vi "Stop Core.vi"(10 "final error code":i32, 11 "TestStand Controller in":refnum<class "Controller API.lvclass">) -> (3 "TestStand Controller out":refnum<class "Controller API.lvclass">)   [LabVIEW 2026, in "Controller API.lvlib" / "Controller API.lvclass"]
uses:
  Controller API.lvclass
  framework/Results/Results.lvclass
  Controller API.lvclass/Controller API.ctl
  framework/Controller/Controller.lvclass
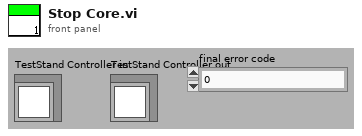
[diagram p1: front panel]
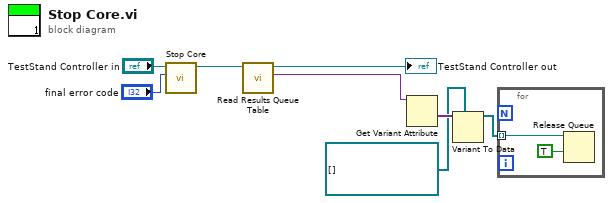
[diagram p0: block diagram]
diagram:
  n1 = call-parent "Stop Core.vi"("final error code"="final error code", "Controller in"="TestStand Controller in") -> ("Controller out"=w6:refnum<class "Controller API.lvclass">)  [unwired: 9 in]
  n2 = call "Read Results Queue Table.vi"("TestStand Controller in"=w6) -> ("Results Queue Table"=w4:variant, "TestStand Controller out"=→"TestStand Controller out":refnum<class "Controller API.lvclass">)  [unwired: 8 in, 1 out]
  n3 = Get Variant Attribute(Variant=w4) -> (values=w2:variant[])  [unwired: 3 in, 3 out]
  n4 = Variant To Data(type=refnum<queue>[] [], Variant=w2) -> (data=w3:refnum<queue>[])  [unwired: 1 in, 1 out]
  n5 = for {
    tunnel: w3 -> [w10] mode=indexing
    n6 = Release Queue(queue=w10, force destroy? (F)=TRUE) -> ()  [unwired: 1 in, 3 out]
  }
